vi "PLC-Setup.vi"(8 "error in":errorcluster, 11 "Idx":i32) -> (0 "error out":errorcluster)   [LabVIEW 2016]
uses:
  PLC.Action.ctl
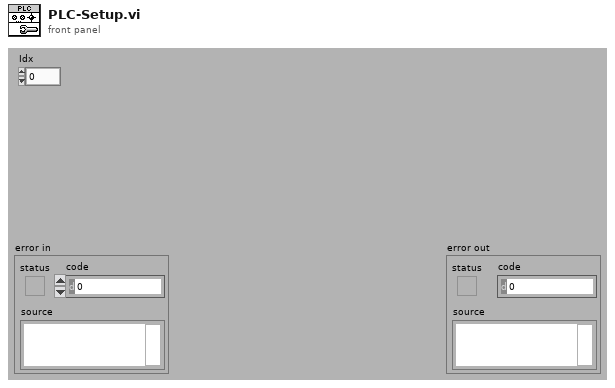
[diagram p1: front panel]
types:
  T1 = typedef "PLC.Action.ctl" = enum32{"idle", "constructor", "destructor", "-- PLC --", "Setup", "NewData", "ChangeOver", "CheckStatus"}
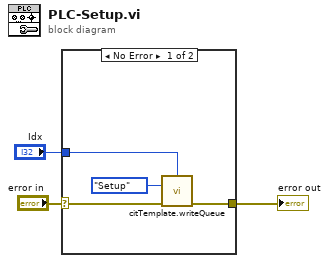
[diagram p0: block diagram]
diagram:
  n1 = case shown="No Error" "error in" {
    selector: "error in" -> [w7 w8]
    tunnel: [w6 w8] -> w2
    tunnel: "Idx" -> [w4 _]
    frame No Error {
      n2 = call "citTemplate.writeQueue.vi"("instance (0)"=w4, "event in (if not connected:all statemachine with data event)"=PLC.Action."Setup" ("Action"), "error in (no error)"=w7) -> ("error out"=w6:errorcluster)  [unwired: 12 in]
    }
    frame Error {
    }
  }
  "error out" <- w2
